vi "Get ISO Timestring.vi"() -> (3 "date/time string":string)   [LabVIEW 2019, in "Acquisition Example.lvlib"]
uses:
  Acquisition Example.lvlib
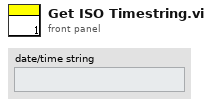
[diagram p1: front panel]
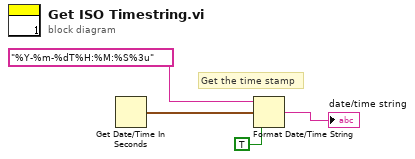
[diagram p0: block diagram]
diagram:
  # "Get the time stamp"
  n1 = Get Date/Time In Seconds() -> (seconds since 1Jan1904=w2:timestamp)
  n2 = Format Date/Time String(time format string (%c)="%Y-%m-%dT%H:%M:%S%3u", seconds (now)=w2, UTC format=TRUE ("want seconds? (F)")) -> (date/time string=→"date/time string":string)
